vi "Sound_Out_16b_mono.vi"(8 "error in (no error)":errorcluster, 10 "Audio Waveform Init":waveform(dbl), 11 "task ID out in":u32) -> (0 "error out":errorcluster, 3 "task ID out out":u32)   [LabVIEW 2011]
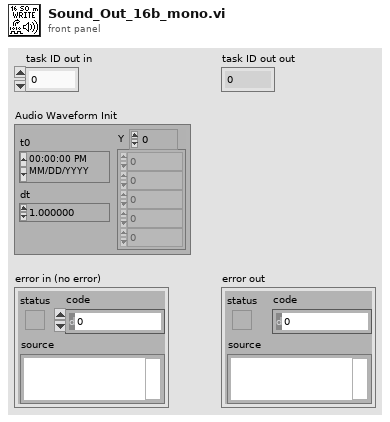
[diagram p1: front panel]
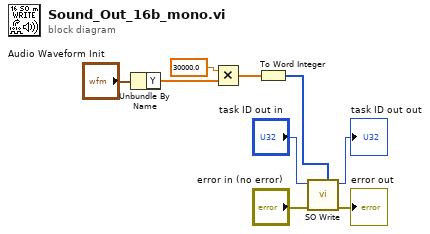
[diagram p0: block diagram]
diagram:
  n1 = Unbundle By Name("Audio Waveform Init") -> ("Y"=w6:dbl[])
  n2 = Multiply(x=30000.0, y=w6) -> (x*y=w7:dbl[])
  n3 = To Word Integer(number=w7) -> (16bit integer=w3:i16[])
  n4 = call <vilib>:"SO Write.vi"("mono 16-bit"=w3, "error in (no error)"="error in (no error)", "task ID in"="task ID out in") -> ("error out"=→"error out":errorcluster, "task ID out"=→"task ID out out":u32)  [unwired: 7 in]
